vi "util_is_in_array.vi"(1 "Array":dbl[](array[numeric]), 2 "Numeric":dbl format="%#_13g") -> (0 "Position":i32)   [LabVIEW 2016]
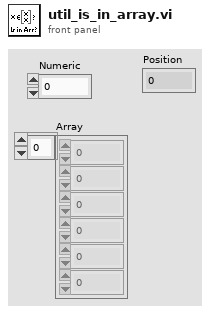
[diagram p1: front panel]
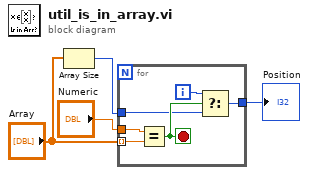
[diagram p0: block diagram]
diagram:
  n1 = Array Size(array="Array") -> (size(s)=w2:i32)
  n2 = for {
    tunnel: "Array" -> [w9] mode=indexing
    tunnel: "Numeric" -> [w10]
    tunnel: w2 -> [w5]
    tunnel: [w7] -> w1
    i -> [w8]
    stop <- w6 stop-if-true
    n3 = Equal?(x=w10, y=w9) -> (x = y?=w6:bool)
    n4 = Select(t=w8, s=w6, f=w5) -> (s? t:f=w7:i32)
  }
  "Position" <- w1
